vi "Temperature Warnings.vi"(8 "Error In":errorcluster, 9 "Min Temperature":dbl, 10 "Max Temperature":dbl, 11 "Current Temperature":dbl) -> (0 "Error Out":errorcluster, 2 "Warning Text":string="No Warning", 3 "Warning?":bool)   [LabVIEW 2015]
doc: "This VI is used to determine the string to output to the weather station based on the current temperature and limit settings.\n\nInputs: Current Temperature (DBL), Minimum Temperature (DBL), and Maximum Temperature (DBL).\nOutputs: Warning Text (string) and Warning? (Boolean)."
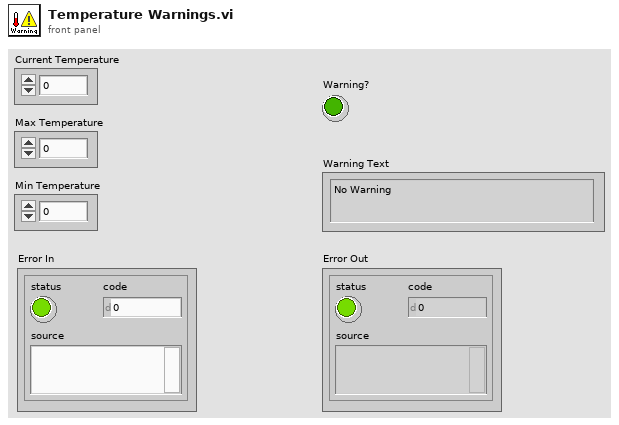
[diagram p1: front panel]
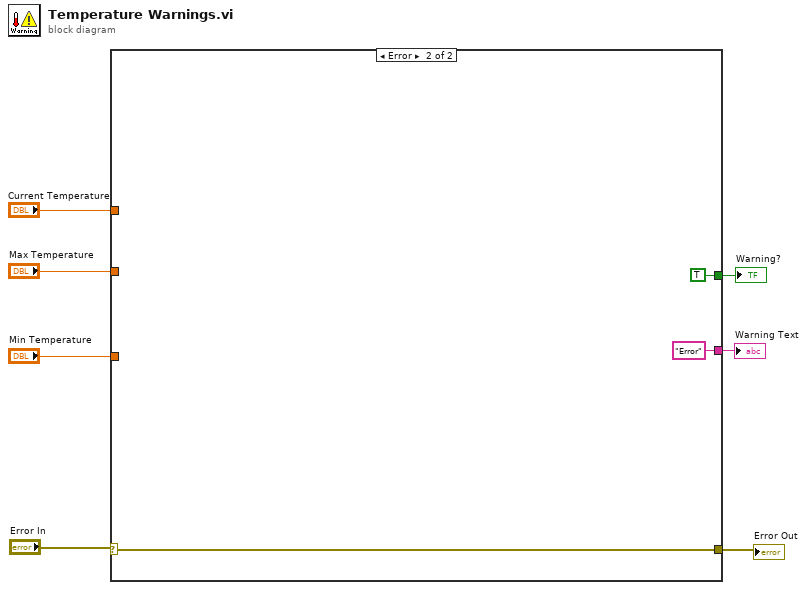
[diagram p0: block diagram]
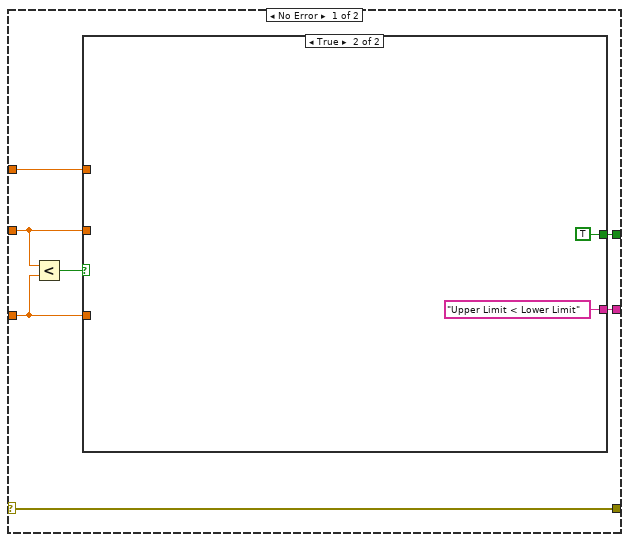
[diagram p2: hidden frame]
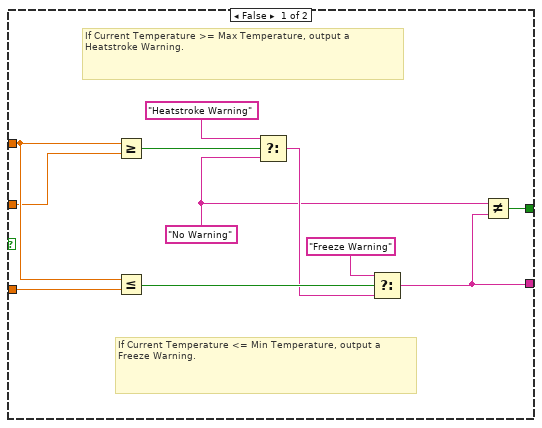
[diagram p3: hidden frame]
diagram:
  n1 = case shown="Error" "Error In" {
    selector: "Error In" -> [w8 w30]
    tunnel: "Current Temperature" -> [w14 _]
    tunnel: [w13 TRUE] -> w6
    tunnel: [w12 "Error" ("f")] -> w5
    tunnel: "Max Temperature" -> [w11 _]
    tunnel: "Min Temperature" -> [w10 _]
    tunnel: [w8 w30] -> w1
    frame No Error {
      n2 = Less?(x=w11, y=w10) -> (x < y?=w9:bool)
      n3 = case shown="True" w9 {
        tunnel: w14 -> [w25 _]
        tunnel: [w24 TRUE] -> w13
        tunnel: [w23 "Upper Limit < Lower Limit" ("f")] -> w12
        tunnel: w11 -> [w16 _]
        tunnel: w10 -> [w15 _]
        frame False {
          w17 = "No Warning" ("f")
          # "If Current Temperature >= Max Temperature, output a Heatstroke Warning."
          # "If Current Temperature <= Min Temperature, output a Freeze Warning."
          n4 = Greater Or Equal?(x=w25, y=w16) -> (x >= y?=w22:bool)
          n5 = Less Or Equal?(x=w25, y=w15) -> (x <= y?=w19:bool)
          n6 = Select(t="Heatstroke Warning", s=w22, f=w17) -> (s? t:f=w18:string)
          n7 = Select(t="Freeze Warning", s=w19, f=w18) -> (s? t:f=w23:string)
          n8 = Not Equal?(x=w17, y=w23) -> (x != y?=w24:bool)
        }
        frame True {
        }
      }
    }
    frame Error {
    }
  }
  "Warning?" <- w6
  "Warning Text" <- w5
  "Error Out" <- w1
